vi "Build2DParamArray.vi"(9 "Step Sizes":dbl[](array[numeric]), 10 "Final Values":dbl[](array[numeric]), 11 "Initial Values":dbl[](array[numeric])) -> (2 "Parameter Array":dbl[][](array[numeric]))   [LabVIEW 2016]
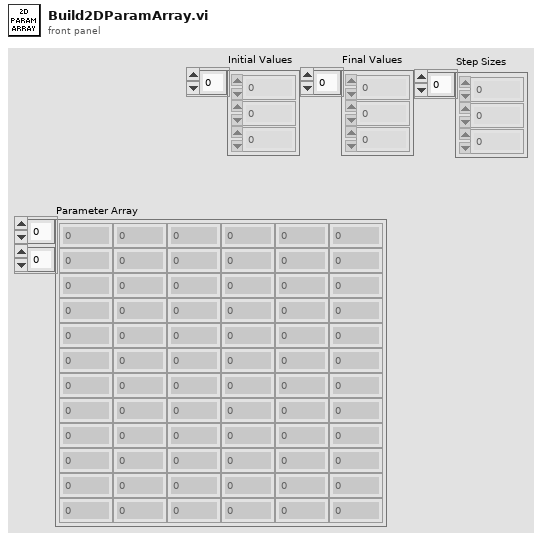
[diagram p1: front panel]
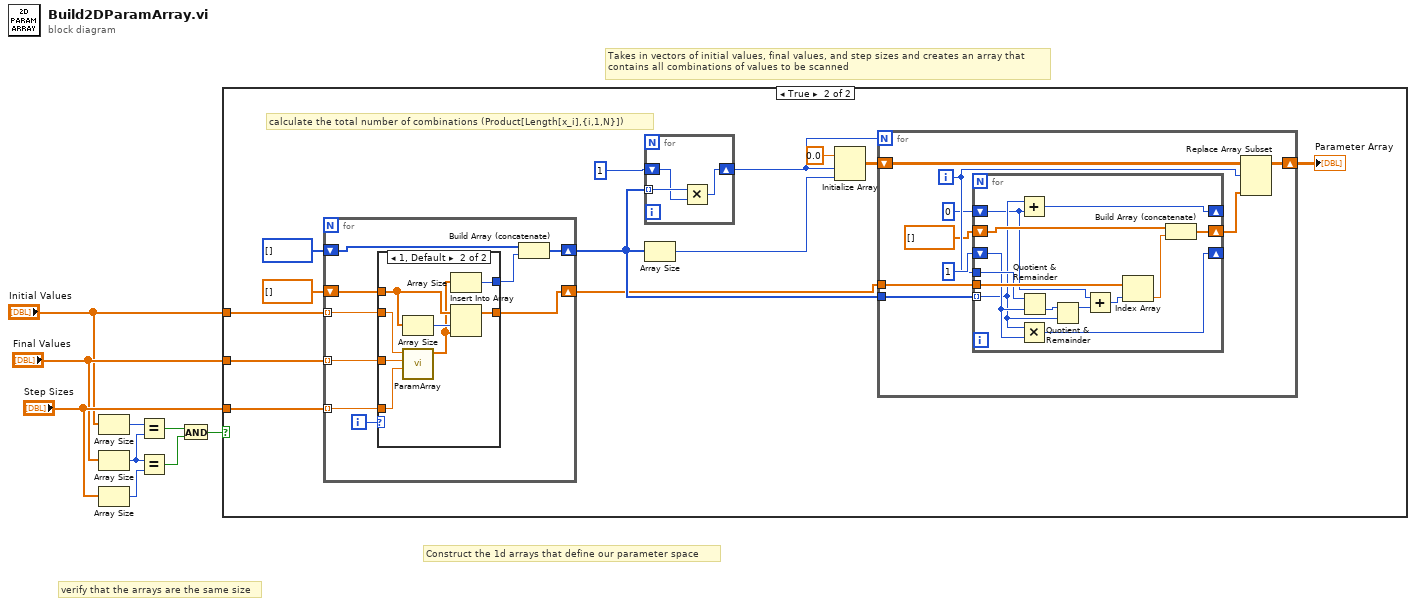
[diagram p0: block diagram]
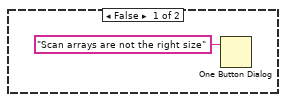
[diagram p2: hidden frame]
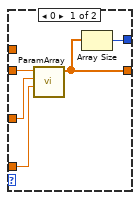
[diagram p3: hidden frame]
diagram:
  # "Construct the 1d arrays that define our parameter space"
  # "Takes in vectors of initial values, final values, and step sizes and creates an array that\ncontains all combinations of values to be scanned"
  # "verify that the arrays are the same size"
  n1 = Array Size(array="Initial Values") -> (size(s)=w7:i32)
  n2 = Array Size(array="Final Values") -> (size(s)=w8:i32)
  n3 = Array Size(array="Step Sizes") -> (size(s)=w9:i32)
  n4 = Equal?(x=w7, y=w8) -> (x = y?=w6:bool)
  n5 = Equal?(x=w8, y=w9) -> (x = y?=w5:bool)
  n6 = And(x=w6, y=w5) -> (x .and. y?=w4:bool)
  n7 = case shown="True" w4 {
    tunnel: "Step Sizes" -> [_ w23]
    tunnel: "Final Values" -> [_ w22]
    tunnel: "Initial Values" -> [_ w21]
    frame False {
      n8 = One Button Dialog(message="Scan arrays are not the right size") -> ()  [unwired: 1 in, 1 out]
    }
    frame True {
      # "calculate the total number of combinations (Product[Length[x_i],{i,1,N}])"
      n9 = for {
        tunnel: w23 -> [w57] mode=indexing
        tunnel: w22 -> [w56] mode=indexing
        tunnel: w21 -> [w55] mode=indexing
        shift-right: [w50] -> w14
        shift-left: dbl[] [] ("Array") -> [w49]
        shift-right: [w52] -> w15
        shift-left: i32[] [] -> [w53]
        i -> [w51]
        n10 = case shown="1, Default" w51 {
          tunnel: w57 -> [w62 w68]
          tunnel: w56 -> [w61 w69]
          tunnel: w55 -> [w60 w70]
          tunnel: [w58 w65] -> w50
          tunnel: [w59 w63] -> w54
          tunnel: w49 -> [_ w67]
          frame 0 {
            n11 = call "ParamArray.vi"("Step Size"=w62, "Final Value"=w61, "Initial Value"=w60) -> ("Array"=w58:dbl[])  [unwired: 8 in]
            n12 = Array Size(array=w58) -> (size(s)=w59:i32)
          }
          frame 1, Default {
            n13 = Array Size(array=w67) -> (size(s)=w66:i32)
            n14 = call "ParamArray.vi"("Step Size"=w68, "Final Value"=w69, "Initial Value"=w70) -> ("Array"=w64:dbl[])  [unwired: 8 in]
            n15 = Array Size(array=w64) -> (size(s)=w63:i32)
            n16 = Insert Into Array(array=w67, index=w66, new element=w64) -> (w65:dbl[])
          }
        }
        n17 = Build Array (concatenate)(w53, w54) -> (w52:i32[])
      }
      n18 = for {
        tunnel: w15 -> [w48] mode=indexing
        shift-right: [w47] -> w17
        shift-left: 1 -> [w46]
        n19 = Multiply(x=w48, y=w46) -> (x*y=w47:i32)
      }
      n20 = Array Size(array=w15) -> (size(s)=w20:i32)
      n21 = Initialize Array(0.0 ("element"), w17, w20) -> (w16:dbl[][])
      n22 = for {
        N: w17 -> [_]
        shift-right: [w31] -> w11
        shift-left: w16 -> [w32]
        tunnel: w15 -> [w30]
        tunnel: w14 -> [w28]
        i -> [w27]
        n23 = for {
          tunnel: w30 -> [w37] mode=indexing
          shift-right: [w45] -> _
          shift-left: 1 -> [w38]
          tunnel: w28 -> [w44]
          tunnel: w27 -> [w43]
          shift-right: [w39] -> w26
          shift-left: dbl[] [] -> [w40]
          shift-right: [w36] -> _
          shift-left: 0 -> [w35]
          n24 = Add(x=w37, y=w35) -> (x+y=w36:i32)
          n25 = Multiply(x=w37, y=w38) -> (x*y=w45:i32)
          n26 = Quotient & Remainder(x=w43, y=w38) -> (floor(x/y)=w42:i32)  [unwired: 1 out]
          n27 = Quotient & Remainder(x=w42, y=w37) -> (x-y*floor(x/y)=w34:i32)  [unwired: 1 out]
          n28 = Add(x=w35, y=w34) -> (x+y=w33:i32)
          n29 = Index Array(array=w44, index=w33) -> (element=w41:dbl)
          n30 = Build Array (concatenate)(w40, w41) -> (w39:dbl[])
        }
        n31 = Replace Array Subset(array=w32, new element=w26, index (row)=w27) -> (w31:dbl[][])  [unwired: 1 in]
      }
      "Parameter Array" <- w11
    }
  }
